vi "Actor Core.vi"(8 "error in":errorcluster, 11 "IMAQdx Actor in":refnum<class "IMAQdx Actor.lvclass">) -> (0 "error out":errorcluster, 3 "Actor out":refnum<class "Actor.lvclass">)   [LabVIEW 2014, in "IMAQdx Actor.lvlib" / "IMAQdx Actor.lvclass"]
doc: "(<B>Filename</B>: Actor Framework.lvlib:Actor.lvclass:Actor Core.vi)\n\nReceives messages to the actor, reacts to them, and initiates any error handling that may shut the actor down.\n\nDescendant classes may override this VI to append parallel tasks for the actor to complete while it handles messages. Overrides use the Call Parent Method node."
uses:
  IMAQdx Actor.lvclass
  <vilib>/ActorFramework/Actor/Actor.lvclass
  Operation Mode.ctl
  <vilib>/userdefined/High Color/IMAQdx.ctl
  <vilib>/vision/Image Controls.llb/IMAQ Image.ctl
  IMAQdx Actor.lvclass/IMAQdx Actor.ctl
  <vilib>/ActorFramework/Actor/Actor.lvclass/Actor.ctl
  <vilib>/ActorFramework/Message Enqueuer/Message Enqueuer.lvclass/Message Enqueuer.ctl
  Camera Actor/Camera Actor Messages/Publish Image Msg/Publish Image Msg.lvclass/Publish Image Msg.ctl
  <vilib>/ActorFramework/Message Enqueuer/Init from Existing Queue.vi
  <vilib>/ActorFramework/Message Enqueuer/Enqueue.vi
  <vilib>/ActorFramework/Message Priority Queue/Priority Enqueue.vi
  Camera Actor/Camera Actor/Camera Actor.lvclass
  <vilib>/ActorFramework/Message Enqueuer/Message Enqueuer.lvclass
  Camera Actor/Camera Actor Messages/Publish Image Msg/Publish Image Msg.lvclass
  IMAQdx Actor.lvlib
  <vilib>/vision/driver/NI_Vision_Acquisition_Software.lvlib
panel:
  in  "Image":T1
  in  "Session In":T2 caption="Session"
  in  "Mode":T3=enum."Break"
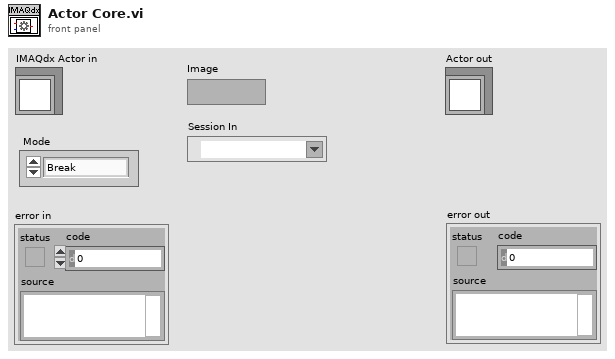
[diagram p1: front panel]
types:
  T1 = typedef "IMAQ Image.ctl" = refnum<image>
  T2 = typedef "IMAQdx.ctl" = refnum<k21>
  T3 = typedef "IMAQdx Actor.lvlib/Operation Mode.ctl" = enum16{"Acquisition", "Break", "Exit"}
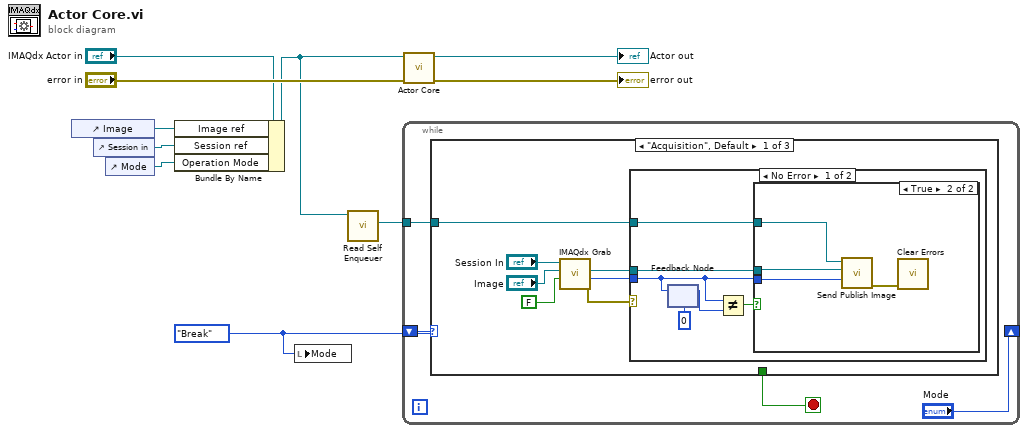
[diagram p0: block diagram]
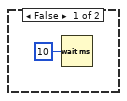
[diagram p2: hidden frame]
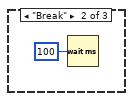
[diagram p4: hidden frame]
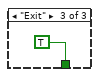
[diagram p5: hidden frame]
diagram:
  w3 = Operation_Mode."Break" ("Operation Mode")
  n1 = control-ref of="Image"() -> (w5:refnum<vi>)
  n2 = control-ref of="Session in"() -> (w4:refnum<vi>)
  n3 = control-ref of="Mode"() -> (w6:refnum<vi>)
  n4 = Bundle By Name(cluster="IMAQdx Actor in", "Image ref"=w5, "Session ref"=w4, "Operation Mode"=w6) -> (w2:refnum<class "IMAQdx Actor.lvclass">)
  n5 = local write "Mode"(w3) -> ()
  n6 = call <vilib>:"Read Self Enqueuer.vi"("Actor"=w2) -> ("Self Enqueuer"=w1:refnum<class "Message Enqueuer.lvclass">)  [unwired: 10 in]
  n7 = while {
    shift-right: ["Mode"] -> _
    shift-left: w3 -> [w14]
    tunnel: w1 -> [w11]
    stop <- w13 stop-if-true
    n8 = case shown="\"Acquisition\", Default" w14 {
      tunnel: [_ _ TRUE ("Value (Signaling)")] -> w13
      tunnel: w11 -> [w17 _ _]
      frame "Acquisition", Default {
        n9 = call <vilib>:"IMAQdx Grab.vi"("Wait for Next Buffer? (Yes)"=FALSE, "Image In"="Image", "Session In"="Session In") -> ("error out"=w15:errorcluster, "Buffer Number Out"=w16:u32, "Image Out"=w18:T1)  [unwired: 5 in, 1 out]
        n10 = case shown="No Error" w15 {
          tunnel: w18 -> [w24 _]
          tunnel: w17 -> [w23 _]
          tunnel: w16 -> [w22 _]
          frame No Error {
            n11 = feedback #1(u32 0 ("Buffer Number Out")) -> (w26:u32)
            n12 = feedback-in #1(w22) -> ()
            n13 = Not Equal?(x=w22, y=w26) -> (x != y?=w25:bool)
            n14 = case shown="True" w25 {
              tunnel: w24 -> [_ w29]
              tunnel: w23 -> [_ w32]
              tunnel: w22 -> [_ w31]
              frame False {
                n15 = Wait (ms)(milliseconds to wait=u32 10) -> ()  [unwired: 1 out]
              }
              frame True {
                n16 = call "Send Publish Image.vi"("Buffer Number"=w31, "Image"=w29, "Message Enqueuer"=w32) -> ("error out"=w30:errorcluster)  [unwired: 7 in, 1 out]
                n17 = call <vilib>:"Clear Errors.vi"("error in (no error)"=w30) -> ()  [unwired: 5 in, 2 out]
              }
            }
          }
          frame Error {
          }
        }
      }
      frame "Break" {
        n18 = Wait (ms)(milliseconds to wait=u32 100) -> ()  [unwired: 1 out]
      }
      frame "Exit" {
      }
    }
  }
  n19 = call-parent "Actor Core.vi"("error in"="error in", "Actor in"=w2) -> ("error out"=→"error out":errorcluster, "Actor out"=→"Actor out":refnum<class "Actor.lvclass">)  [unwired: 8 in]
